vi "File - two files distinct roots.vi"(8 "error in (no error)":errorcluster) -> (0 "error out":errorcluster)   [LabVIEW 2026, in "Tests.lvlib"]
doc: "Integration test (Caraya). Verifies a statement logged through the Logger reaches a single registered appender. Launches a manager with the default file disabled and a queue-mode relay capture probe (Open Test Mgr), logs one INFO statement, dequeues from the capture queue with a timeout, and asserts it was delivered and its message matches. Tears down with Close Test Mgr regardless of assertion outcome (SRS-LMBR-019). Uses the manager fixture; no temp root needed.\n\nImplements LMBR-T-029 -> SRS-019. Assert-level IDs: Test-ID-Assert-Checklist.md."
uses:
  Tests.lvlib
  src/TypeDefs/Severity.ctl
  src/TypeDefs/FileAppenderConfig.ctl
  src/TypeDefs/AppenderConfig.ctl
  src/TypeDefs/Filter.ctl
  src/TypeDefs/FilterMode.ctl
  src/TypeDefs/DropPolicy.ctl
  src/TypeDefs/FileConfig.ctl
  <vilib>/addons/_JKI Toolkits/Caraya/classes/Assert/Assert Equal Value_Variant.vi
  <vilib>/addons/_JKI Toolkits/Caraya/classes/Assert/Assert True.vi
  <vilib>/addons/_JKI Toolkits/Caraya/classes/Assert/Assert False.vi
  <vilib>/addons/_JKI Toolkits/Caraya/classes/Test/Test.lvclass
  src/Lumberjack.lvlib
  src/Public/Logger.lvclass/Logger.lvclass
  <vilib>/addons/_JKI Toolkits/Caraya/classes/Assert/Assert.lvclass
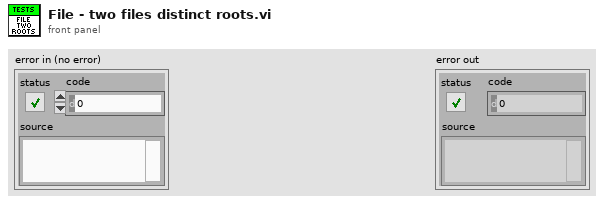
[diagram p1: front panel]
types:
  T1 = typedef "Lumberjack.lvlib/Severity.ctl" = enum16{"OFF", "FATAL", "ERROR", "WARN", "INFO", "DEBUG", "TRACE", "ALL"}
  T2 = typedef "Lumberjack.lvlib/FileAppenderConfig.ctl" = cluster{"common":T3, "file":T7}
  T3 = typedef "Lumberjack.lvlib/AppenderConfig.ctl" = cluster{"id":string, "threshold":T1, "filter":T4, "queueBound":i32, "dropPolicy":T6, "useUTC":bool}
  T4 = typedef "Lumberjack.lvlib/Filter.ctl" = cluster{"mode":T5, "levelMin":T1, "levelMax":T1, "tagPrefix":string}
  T5 = typedef "Lumberjack.lvlib/FilterMode.ctl" = enum16{"Mirror", "Routed"}
  T6 = typedef "Lumberjack.lvlib/DropPolicy.ctl" = enum16{"DropOldest", "DropNewest", "LevelAware"}
  T7 = typedef "Lumberjack.lvlib/FileConfig.ctl" = cluster{"rootFolder":path, "maxFileSize":i64, "maxFileCount":i32, "baseName":string, "extension":string, "delimiter":string, "calendarFolderTree":bool}
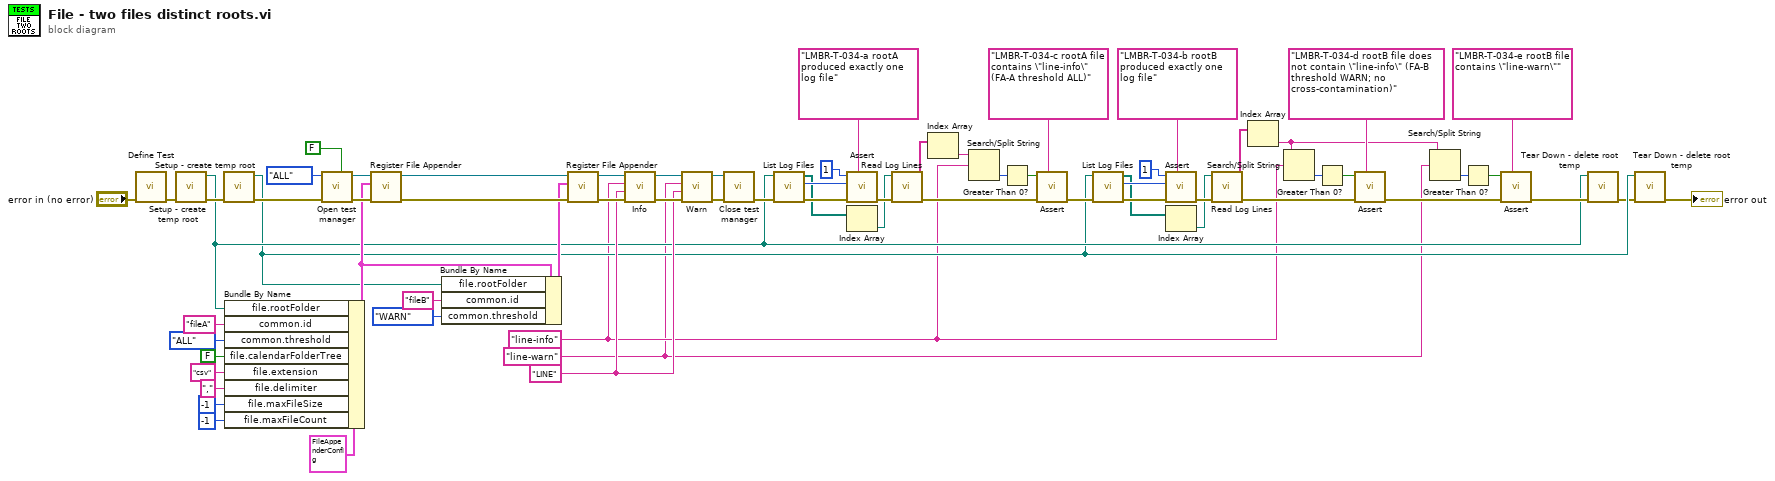
[diagram p0: block diagram]
diagram:
  w45 = "LINE" ("sourceTag")
  w3 = "line-warn" ("message")
  w4 = "line-info" ("message")
  n1 = call <vilib>:"Define Test.vi"("error in (no error)"="error in (no error)") -> ("error out"=w66:errorcluster)  [unwired: 9 in, 1 out]
  n2 = call "Setup - create temp root.vi"("error in (no error)"=w66) -> ("error out"=w65:errorcluster, "tempRoot"=w9:path)  [unwired: 9 in]
  n3 = call "Setup - create temp root.vi"("error in (no error)"=w65) -> ("error out"=w64:errorcluster, "tempRoot"=w8:path)  [unwired: 9 in]
  n4 = Bundle By Name(cluster=T2 {"common"={"id"="", "threshold"=enum."INFO", "filter"={"mode"=enum."Mirror", "levelMin"=enum."INFO", "levelMax"=enum."INFO", "tagPrefix"=""}, "queueBound"=0, "dropPolicy"=enum."DropOldest", "useUTC"=FALSE}, "file"={"rootFolder"=path "", "maxFileSize"=0, "maxFileCount"=0, "baseName"="", "extension"="", "delimiter"="", "calendarFolderTree"=FALSE}} ("FileAppenderConfig"), "file.rootFolder"=w9, "common.id"="fileA", "common.threshold"=Severity."ALL", "file.calendarFolderTree"=FALSE, "file.extension"="csv", "file.delimiter"=",", "file.maxFileSize"=i64 -1, "file.maxFileCount"=-1) -> (w58:T2)
  n5 = call "Open test manager.vi"("enableDefaultFile"=FALSE, "error in (no error)"=w64, "globalThreshold"=Severity."ALL") -> ("error out"=w62:errorcluster, "Logger out"=w57:refnum<class "Logger.lvclass">)  [unwired: 7 in]
  n6 = call "Register File Appender.vi"("error in (no error)"=w62, "FileAppenderConfig"=w58, "Logger in"=w57) -> ("error out"=w61:errorcluster, "Logger out"=w56:refnum<class "Logger.lvclass">)  [unwired: 6 in, 1 out]
  n7 = Bundle By Name(cluster=w58, "file.rootFolder"=w8, "common.id"="fileB", "common.threshold"=Severity."WARN") -> (w52:T2)
  n8 = call "Register File Appender.vi"("error in (no error)"=w61, "FileAppenderConfig"=w52, "Logger in"=w56) -> ("error out"=w50:errorcluster, "Logger out"=w51:refnum<class "Logger.lvclass">)  [unwired: 6 in, 1 out]
  n9 = call "Info.vi"("error in (no error)"=w50, "sourceTag"=w45, "message"=w4, "Logger in"=w51) -> ("error out"=w49:errorcluster, "Logger out"=w48:refnum<class "Logger.lvclass">)  [unwired: 6 in]
  n10 = call "Warn.vi"("error in (no error)"=w49, "sourceTag"=w45, "message"=w3, "Logger in"=w48) -> ("error out"=w47:errorcluster, "Logger out"=w46:refnum<class "Logger.lvclass">)  [unwired: 6 in]
  n11 = call "Close test manager.vi"("error in (no error)"=w47, "Logger in"=w46) -> ("error out"=w44:errorcluster)  [unwired: 7 in]
  n12 = call "List Log Files.vi"("error in (no error)"=w44, "rootFolder"=w9) -> ("error out"=w42:errorcluster, "count"=w43:i32, "filePaths"=w41:path[])  [unwired: 7 in]
  n13 = call-poly <vilib>:"Assert.vi"("Label"="LMBR-T-034-a rootA produced exactly one log file", "error in (no error)"=w42, "Actual"=w43, "Expected"=1) -> ("error out"=w20:errorcluster)  [unwired: 6 in, 1 out]
  n14 = Index Array(array=w41) -> (element=w18:path)  [unwired: 1 in]
  n15 = call "Read Log Lines.vi"("error in (no error)"=w20, "filePath"=w18) -> ("error out"=w19:errorcluster, "lines"=w7:string[])  [unwired: 8 in]
  n16 = Index Array(array=w7) -> (element=w6:string)  [unwired: 1 in]
  n17 = Search/Split String(string=w6, search string/char (-)=w4) -> (offset of match=w39:i32)  [unwired: 1 in, 2 out]
  n18 = Greater Than 0?(x=w39) -> (x > 0?=w38:bool)
  n19 = call-poly <vilib>:"Assert.vi"("Label"="LMBR-T-034-c rootA file contains \"line-info\" (FA-A threshold ALL)", "error in (no error)"=w19, "True?"=w38) -> ("error out"=w31:errorcluster)  [unwired: 7 in, 1 out]
  n20 = call "List Log Files.vi"("error in (no error)"=w31, "rootFolder"=w8) -> ("error out"=w36:errorcluster, "count"=w37:i32, "filePaths"=w35:path[])  [unwired: 7 in]
  n21 = call-poly <vilib>:"Assert.vi"("Label"="LMBR-T-034-b rootB produced exactly one log file", "error in (no error)"=w36, "Actual"=w37, "Expected"=1) -> ("error out"=w17:errorcluster)  [unwired: 6 in, 1 out]
  n22 = Index Array(array=w35) -> (element=w15:path)  [unwired: 1 in]
  n23 = call "Read Log Lines.vi"("error in (no error)"=w17, "filePath"=w15) -> ("error out"=w16:errorcluster, "lines"=w5:string[])  [unwired: 8 in]
  n24 = Index Array(array=w5) -> (element=w2:string)  [unwired: 1 in]
  n25 = Search/Split String(string=w2, search string/char (-)=w4) -> (offset of match=w33:i32)  [unwired: 1 in, 2 out]
  n26 = Greater Than 0?(x=w33) -> (x > 0?=w32:bool)
  n27 = call-poly <vilib>:"Assert.vi"("Label"="LMBR-T-034-d rootB file does not contain \"line-info\" (FA-B threshold WARN; no cross-contamination)", "error in (no error)"=w16, "False?"=w32) -> ("error out"=w27:errorcluster)  [unwired: 7 in, 1 out]
  n28 = Search/Split String(string=w2, search string/char (-)=w3) -> (offset of match=w29:i32)  [unwired: 1 in, 2 out]
  n29 = Greater Than 0?(x=w29) -> (x > 0?=w28:bool)
  n30 = call-poly <vilib>:"Assert.vi"("Label"="LMBR-T-034-e rootB file contains \"line-warn\"", "error in (no error)"=w27, "True?"=w28) -> ("error out"=w11:errorcluster)  [unwired: 7 in, 1 out]
  n31 = call "Tear Down - delete root temp.vi"("error in (no error)"=w11, "tempRoot"=w9) -> ("error out"=w1:errorcluster)  [unwired: 9 in]
  n32 = call "Tear Down - delete root temp.vi"("error in (no error)"=w1, "tempRoot"=w8) -> ("error out"=→"error out":errorcluster)  [unwired: 9 in]
